vi "EnumArray and Enum.vi"(0 "enum":T6(ring)=enum."a", 1 "ArrayEnums":T5(array[ring])=[enum."a", enum."red", enum."a", enum."a", enum."a", enum."a", enum."red"], 4 "Cluster":T1={"enum"=enum."a", "ArrayEnums"=[]}, 7 "Array 11":T3(array[cluster])=[[{"enum"=enum."a", "ArrayEnums"=[]}, {"enum"=enum."a", "ArrayEnums"=[]}, {"enum"=enum."a", "ArrayEnums"=[]}, {"enum"=enum."a", "ArrayEnums"=[]}, {"enum"=enum."a", "ArrayEnums"=[]}], [{"enum"=enum."a", "ArrayEnums"=[]}, {"enum"=enum."a", "ArrayEnums"=[]}, {"enum"=enum."a", "ArrayEnums"=[]}, {"enum"=enum."a", "ArrayEnums"=[]}, {"enum"=enum."a", "ArrayEnums"=[]}], [{"enum"=enum."a", "ArrayEnums"=[]}, {"enum"=enum."a", "ArrayEnums"=[]}, {"enum"=enum."a", "ArrayEnums"=[]}, {"enum"=enum."a", "ArrayEnums"=[]}, {"enum"=enum."a", "ArrayEnums"=[]}], [{"enum"=enum."a", "ArrayEnums"=[]}, {"enum"=enum."a", "ArrayEnums"=[]}, {"enum"=enum."a", "ArrayEnums"=[]}, {"enum"=enum."a", "ArrayEnums"=[]}, {"enum"=enum."red", "ArrayEnums"=[enum."a", enum."a", enum."a", enum."a", enum."black"]}]], 14 "Array":T4(array[cluster])=[{"enum"=enum."a", "ArrayEnums"=[]}, {"enum"=enum."a", "ArrayEnums"=[]}, {"enum"=enum."a", "ArrayEnums"=[]}, {"enum"=enum."red", "ArrayEnums"=[enum."a", enum."a", enum."a", enum."a", enum."black"]}], 17 "ClusterinCluster":T2={"Cluster 4"={"enum"=enum."a", "ArrayEnums"=[]}}) -> (3 "ArrayEnums 2":T5(array[ring]), 8 "a 2":T6(ring)=enum."a", 9 "Array 12":T3(array[cluster]), 18 "Cluster 2":T1={"enum"=enum."a", "ArrayEnums"=[]}, 27 "Array 4":T4(array[cluster]))   [LabVIEW 2012]
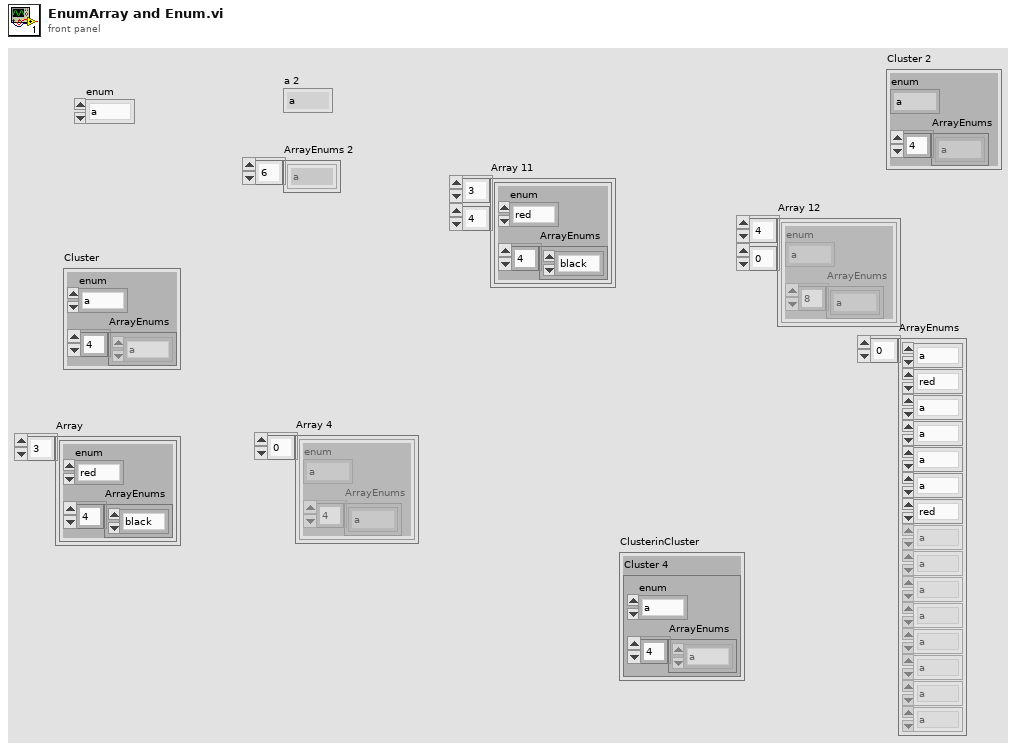
[diagram p1: front panel]
types:
  T1 = cluster{"enum":enum16{"f", "e", "d", "c", "b", "a", "blue", "red", "ffff", "black"}, "ArrayEnums":enum16{"f", "e", "d", "c", "b", "a", "blue", "red", "ffff", "black"}[]}
  T2 = cluster{"Cluster 4":cluster{"enum":enum16{"f", "e", "d", "c", "b", "a", "blue", "red", "ffff", "black"}, "ArrayEnums":enum16{"f", "e", "d", "c", "b", "a", "blue", "red", "ffff", "black"}[]}}
  T3 = cluster{"enum":enum16{"f", "e", "d", "c", "b", "a", "blue", "red", "ffff", "black"}, "ArrayEnums":enum16{"f", "e", "d", "c", "b", "a", "blue", "red", "ffff", "black"}[]}[][]
  T4 = cluster{"enum":enum16{"f", "e", "d", "c", "b", "a", "blue", "red", "ffff", "black"}, "ArrayEnums":enum16{"f", "e", "d", "c", "b", "a", "blue", "red", "ffff", "black"}[]}[]
  T5 = enum16{"f", "e", "d", "c", "b", "a", "blue", "red", "ffff", "black"}[]
  T6 = enum16{"f", "e", "d", "c", "b", "a", "blue", "red", "ffff", "black"}
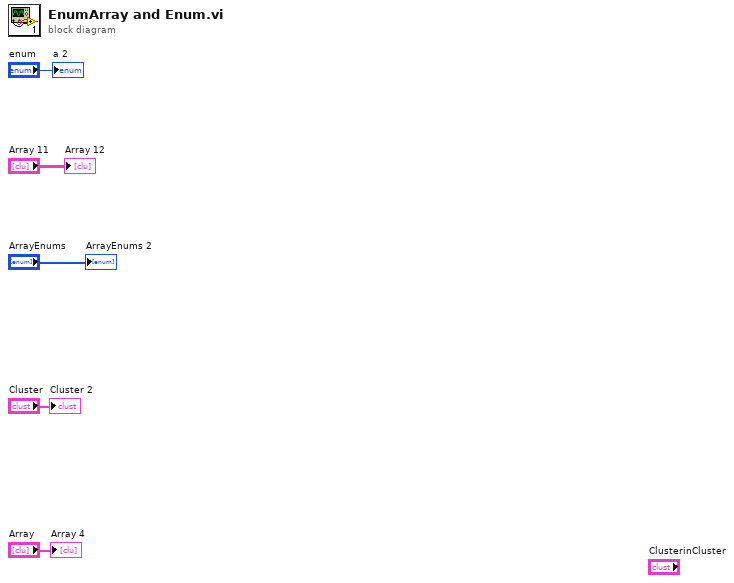
[diagram p0: block diagram]
diagram:
  "a 2" <- "enum"
  "ArrayEnums 2" <- "ArrayEnums"
  "Array 4" <- "Array"
  "Array 12" <- "Array 11"
  "Cluster 2" <- "Cluster"
